vi "SendCerebus32.vi"(1 "String":string, 4 "Mode":T1(ring)) -> ()   [LabVIEW 2013]
uses:
  <vilib>/DAQmx/write.llb/DAQmx Write (Digital 1D Bool 1Chan 1Samp).vi
  <vilib>/DAQmx/miscellaneous.llb/DAQmx Fill In Error Info.vi
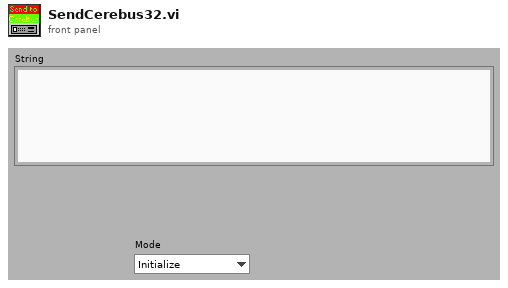
[diagram p1: front panel]
types:
  T1 = enum16{"Initialize", "String", "Start", "New Session", "Stop", "Resume", "Close"}
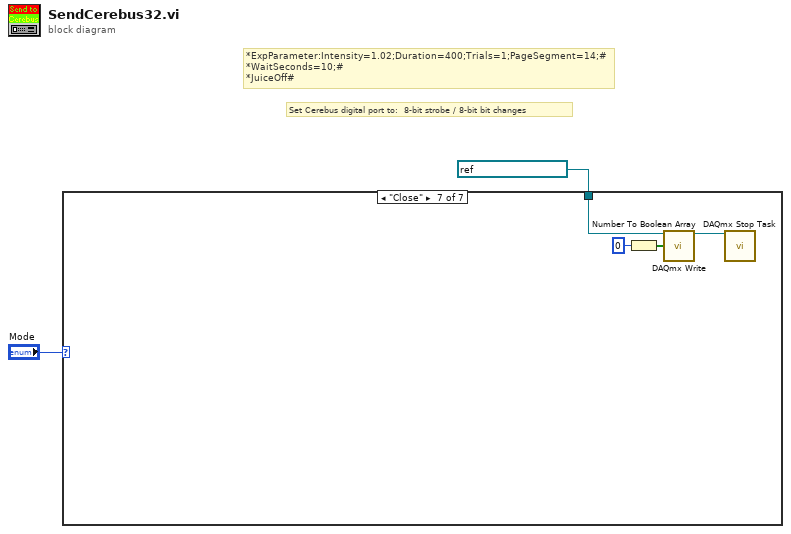
[diagram p0: block diagram]
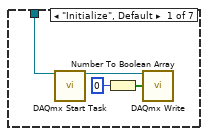
[diagram p2: hidden frame]
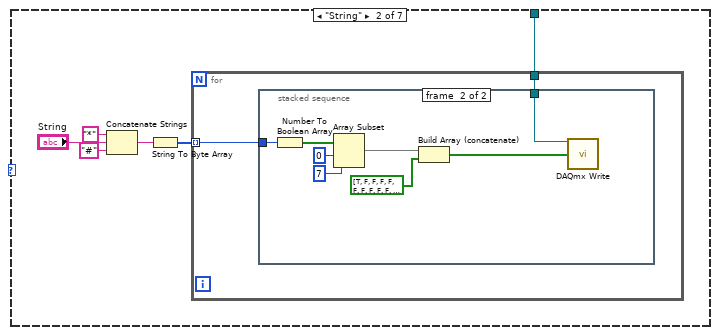
[diagram p3: hidden frame]
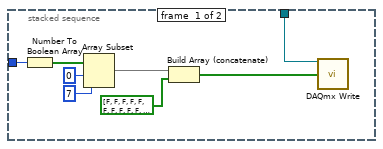
[diagram p4: hidden frame]
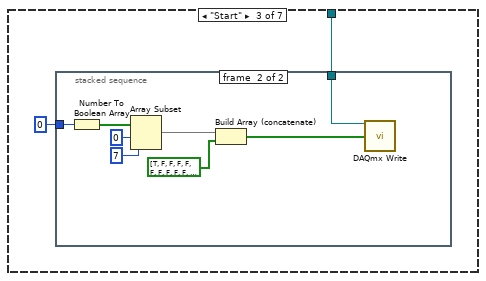
[diagram p5: hidden frame]
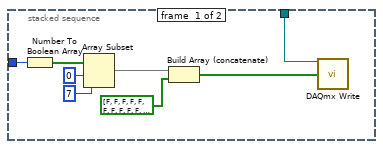
[diagram p6: hidden frame]
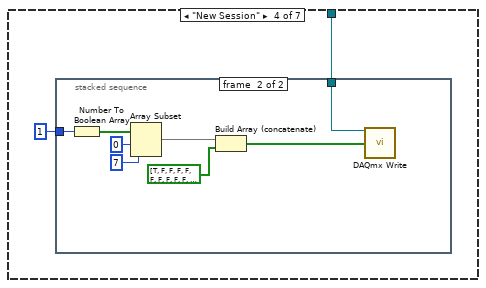
[diagram p7: hidden frame]
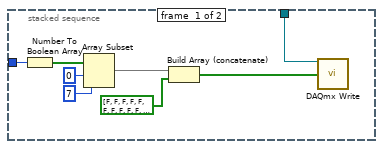
[diagram p8: hidden frame]
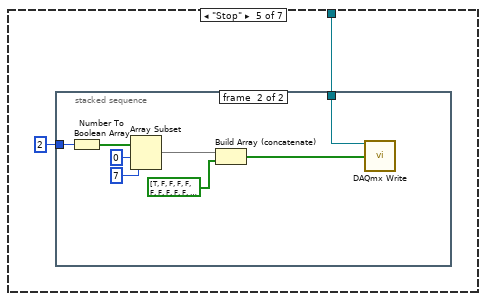
[diagram p9: hidden frame]
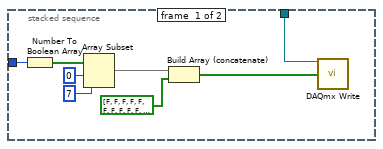
[diagram p10: hidden frame]
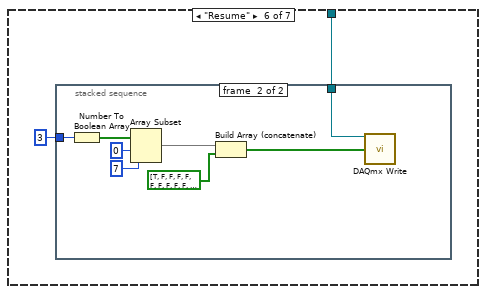
[diagram p11: hidden frame]
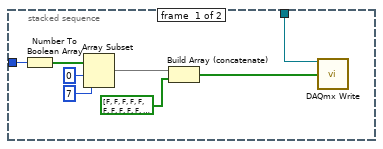
[diagram p12: hidden frame]
diagram:
  # "Set Cerebus digital port to:  8-bit strobe / 8-bit bit changes"
  # "*ExpParameter:Intensity=1.02;Duration=400;Trials=1;PageSegment=14;#\n*WaitSeconds=10;#\n*JuiceOff#"
  n1 = case shown="\"Close\"" "Mode" {
    tunnel: refnum<k21> "cerebus_markers" ("task/channels in") -> [w6 w7 w32 w50 w68 w86 w103]
    frame "Initialize", Default {
      n2 = call <vilib>:"DAQmx Start Task.vi"("task/channels in"=w6) -> ("task out"=w5:refnum<k21>)  [unwired: 13 in, 1 out]
      n3 = Number To Boolean Array(number=u32 0) -> (Boolean array=w3:bool[])
      n4 = call-poly <vilib>:"DAQmx Write.vi"("task/channels in"=w5, "data"=w3) -> ()  [unwired: 11 in, 3 out]
    }
    frame "String" {
      n5 = Concatenate Strings("*", "String", "#" ("string")) -> (w9:string)
      n6 = String To Byte Array(string=w9) -> (unsigned byte array=w12:u8[])
      n7 = for {
        tunnel: w12 -> [w13] mode=indexing
        tunnel: w7 -> [w14]
        n8 = stacked-sequence {
          tunnel: w13 -> [w22 w24]
          tunnel: w14 -> [w21 w30]
          frame #0 {
            n9 = Number To Boolean Array(number=w22) -> (Boolean array=w20:bool[])
            n10 = Array Subset(array=w20, index=0, length=7) -> (w17:bool[])
            n11 = Build Array (concatenate)(w17, bool[] [FALSE, FALSE, FALSE, FALSE, FALSE, FALSE, FALSE, FALSE, FALSE, FALSE, FALSE, FALSE, FALSE, FALSE, FALSE, FALSE, FALSE, FALSE, FALSE, FALSE, FALSE, FALSE, FALSE, FALSE, FALSE] ("array")) -> (w15:bool[])
            n12 = call-poly <vilib>:"DAQmx Write.vi"("task/channels in"=w21, "data"=w15) -> ()  [unwired: 11 in, 3 out]
          }
          frame #1 {
            n13 = Number To Boolean Array(number=w24) -> (Boolean array=w29:bool[])
            n14 = Array Subset(array=w29, index=0, length=7) -> (w26:bool[])
            n15 = Build Array (concatenate)(w26, bool[] [TRUE, FALSE, FALSE, FALSE, FALSE, FALSE, FALSE, FALSE, FALSE, FALSE, FALSE, FALSE, FALSE, FALSE, FALSE, FALSE, FALSE, FALSE, FALSE, FALSE, FALSE, FALSE, FALSE, FALSE, FALSE] ("array")) -> (w23:bool[])
            n16 = call-poly <vilib>:"DAQmx Write.vi"("task/channels in"=w30, "data"=w23) -> ()  [unwired: 11 in, 3 out]
          }
        }
      }
    }
    frame "Start" {
      n17 = stacked-sequence {
        tunnel: u8 0 -> [w40 w42]
        tunnel: w32 -> [w39 w48]
        frame #0 {
          n18 = Number To Boolean Array(number=w40) -> (Boolean array=w38:bool[])
          n19 = Array Subset(array=w38, index=0, length=7) -> (w35:bool[])
          n20 = Build Array (concatenate)(w35, bool[] [FALSE, FALSE, FALSE, FALSE, FALSE, FALSE, FALSE, FALSE, FALSE, FALSE, FALSE, FALSE, FALSE, FALSE, FALSE, FALSE, FALSE, FALSE, FALSE, FALSE, FALSE, FALSE, FALSE, FALSE, FALSE] ("array")) -> (w33:bool[])
          n21 = call-poly <vilib>:"DAQmx Write.vi"("task/channels in"=w39, "data"=w33) -> ()  [unwired: 11 in, 3 out]
        }
        frame #1 {
          n22 = Number To Boolean Array(number=w42) -> (Boolean array=w47:bool[])
          n23 = Array Subset(array=w47, index=0, length=7) -> (w44:bool[])
          n24 = Build Array (concatenate)(w44, bool[] [TRUE, FALSE, FALSE, FALSE, FALSE, FALSE, FALSE, FALSE, FALSE, FALSE, FALSE, FALSE, FALSE, FALSE, FALSE, FALSE, FALSE, FALSE, FALSE, FALSE, FALSE, FALSE, FALSE, FALSE, FALSE] ("array")) -> (w41:bool[])
          n25 = call-poly <vilib>:"DAQmx Write.vi"("task/channels in"=w48, "data"=w41) -> ()  [unwired: 11 in, 3 out]
        }
      }
    }
    frame "New Session" {
      n26 = stacked-sequence {
        tunnel: u8 1 -> [w58 w60]
        tunnel: w50 -> [w57 w66]
        frame #0 {
          n27 = Number To Boolean Array(number=w58) -> (Boolean array=w56:bool[])
          n28 = Array Subset(array=w56, index=0, length=7) -> (w53:bool[])
          n29 = Build Array (concatenate)(w53, bool[] [FALSE, FALSE, FALSE, FALSE, FALSE, FALSE, FALSE, FALSE, FALSE, FALSE, FALSE, FALSE, FALSE, FALSE, FALSE, FALSE, FALSE, FALSE, FALSE, FALSE, FALSE, FALSE, FALSE, FALSE, FALSE] ("array")) -> (w51:bool[])
          n30 = call-poly <vilib>:"DAQmx Write.vi"("task/channels in"=w57, "data"=w51) -> ()  [unwired: 11 in, 3 out]
        }
        frame #1 {
          n31 = Number To Boolean Array(number=w60) -> (Boolean array=w65:bool[])
          n32 = Array Subset(array=w65, index=0, length=7) -> (w62:bool[])
          n33 = Build Array (concatenate)(w62, bool[] [TRUE, FALSE, FALSE, FALSE, FALSE, FALSE, FALSE, FALSE, FALSE, FALSE, FALSE, FALSE, FALSE, FALSE, FALSE, FALSE, FALSE, FALSE, FALSE, FALSE, FALSE, FALSE, FALSE, FALSE, FALSE] ("array")) -> (w59:bool[])
          n34 = call-poly <vilib>:"DAQmx Write.vi"("task/channels in"=w66, "data"=w59) -> ()  [unwired: 11 in, 3 out]
        }
      }
    }
    frame "Stop" {
      n35 = stacked-sequence {
        tunnel: u8 2 -> [w76 w78]
        tunnel: w68 -> [w75 w84]
        frame #0 {
          n36 = Number To Boolean Array(number=w76) -> (Boolean array=w74:bool[])
          n37 = Array Subset(array=w74, index=0, length=7) -> (w71:bool[])
          n38 = Build Array (concatenate)(w71, bool[] [FALSE, FALSE, FALSE, FALSE, FALSE, FALSE, FALSE, FALSE, FALSE, FALSE, FALSE, FALSE, FALSE, FALSE, FALSE, FALSE, FALSE, FALSE, FALSE, FALSE, FALSE, FALSE, FALSE, FALSE, FALSE] ("array")) -> (w69:bool[])
          n39 = call-poly <vilib>:"DAQmx Write.vi"("task/channels in"=w75, "data"=w69) -> ()  [unwired: 11 in, 3 out]
        }
        frame #1 {
          n40 = Number To Boolean Array(number=w78) -> (Boolean array=w83:bool[])
          n41 = Array Subset(array=w83, index=0, length=7) -> (w80:bool[])
          n42 = Build Array (concatenate)(w80, bool[] [TRUE, FALSE, FALSE, FALSE, FALSE, FALSE, FALSE, FALSE, FALSE, FALSE, FALSE, FALSE, FALSE, FALSE, FALSE, FALSE, FALSE, FALSE, FALSE, FALSE, FALSE, FALSE, FALSE, FALSE, FALSE] ("array")) -> (w77:bool[])
          n43 = call-poly <vilib>:"DAQmx Write.vi"("task/channels in"=w84, "data"=w77) -> ()  [unwired: 11 in, 3 out]
        }
      }
    }
    frame "Resume" {
      n44 = stacked-sequence {
        tunnel: u8 3 -> [w94 w96]
        tunnel: w86 -> [w93 w102]
        frame #0 {
          n45 = Number To Boolean Array(number=w94) -> (Boolean array=w92:bool[])
          n46 = Array Subset(array=w92, index=0, length=7) -> (w89:bool[])
          n47 = Build Array (concatenate)(w89, bool[] [FALSE, FALSE, FALSE, FALSE, FALSE, FALSE, FALSE, FALSE, FALSE, FALSE, FALSE, FALSE, FALSE, FALSE, FALSE, FALSE, FALSE, FALSE, FALSE, FALSE, FALSE, FALSE, FALSE, FALSE, FALSE] ("array")) -> (w87:bool[])
          n48 = call-poly <vilib>:"DAQmx Write.vi"("task/channels in"=w93, "data"=w87) -> ()  [unwired: 11 in, 3 out]
        }
        frame #1 {
          n49 = Number To Boolean Array(number=w96) -> (Boolean array=w101:bool[])
          n50 = Array Subset(array=w101, index=0, length=7) -> (w98:bool[])
          n51 = Build Array (concatenate)(w98, bool[] [TRUE, FALSE, FALSE, FALSE, FALSE, FALSE, FALSE, FALSE, FALSE, FALSE, FALSE, FALSE, FALSE, FALSE, FALSE, FALSE, FALSE, FALSE, FALSE, FALSE, FALSE, FALSE, FALSE, FALSE, FALSE] ("array")) -> (w95:bool[])
          n52 = call-poly <vilib>:"DAQmx Write.vi"("task/channels in"=w102, "data"=w95) -> ()  [unwired: 11 in, 3 out]
        }
      }
    }
    frame "Close" {
      n53 = Number To Boolean Array(number=u32 0) -> (Boolean array=w105:bool[])
      n54 = call-poly <vilib>:"DAQmx Write.vi"("task/channels in"=w103, "data"=w105) -> ("task out"=w104:refnum<k21>)  [unwired: 11 in, 2 out]
      n55 = call <vilib>:"DAQmx Stop Task.vi"("task/channels in"=w104) -> ()  [unwired: 13 in, 2 out]
    }
  }
